vi "OD.vi"(2 "error in (no error)":errorcluster caption="错误输入（无错误）", 3 "字符串":string, 4 "路径":path) -> (0 "error out":errorcluster caption="错误输出", 1 "引用句柄输出":refnum<file>)   [LabVIEW 2017]
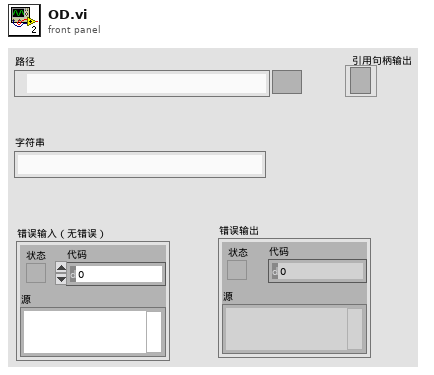
[diagram p1: front panel]
types:
  T1 = enum16{"open", "replace", "create", "open or create", "replace or create", "replace or create with confirmation"}
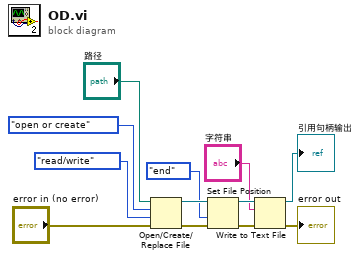
[diagram p0: block diagram]
diagram:
  n1 = Open/Create/Replace File(file path (use dialog)="路径", error in="error in (no error)", operation (0:open)=T1."open or create" ("操作(0:open)"), access (0:read/write)=enum16{"read/write", "read-only", "write-only"}."read/write" ("权限(0:read/write)")) -> (refnum out=w7:refnum<file>, error out=w8:errorcluster)  [unwired: 2 in, 1 out]
  n2 = Set File Position(refnum=w7, from (0:start)=enum16{"start", "end", "current"}."end" ("自（0:起始）"), error in=w8) -> (refnum out=w5:refnum<file>, error out=w4:errorcluster)  [unwired: 1 in]
  n3 = Write to Text File(file (use dialog)=w5, text="字符串", error in=w4) -> (refnum out=→"引用句柄输出":refnum<file>, error out=→"error out":errorcluster)  [unwired: 1 in, 1 out]
